vi "ZMQTestSubscriber.vi"() -> ()   [LabVIEW 2017]
uses:
  <vilib>/addons/zeromq/socket_type.ctl
  <vilib>/addons/zeromq/socket_options.ctl
  <vilib>/Analysis/baseanly.llb/Mean (DBL).vi
  <vilib>/addons/zeromq/zmq_context.lvclass
  <vilib>/addons/zeromq/zeromq.lvlib
  <vilib>/addons/zeromq/zmq_socket.lvclass
  <vilib>/Analysis/NI_AALBase.lvlib
panel:
  out "Full event latency std dev":dbl
  out "Full event latency mean":dbl
  out "Short event latency std dev":dbl
  out "Short event latency mean":dbl
  out "Full event latency (ms)":T1(graph)
  out "Short event latency (ms)":T1(graph)
  in  "port":u16=5560
  in  "Stop Button":bool
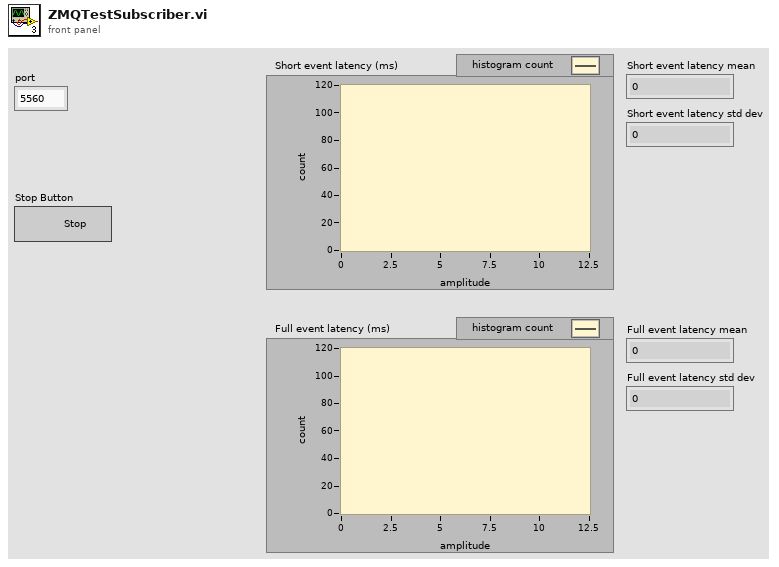
[diagram p1: front panel]
types:
  T1 = cluster{"X Values":dbl[], "Histogram: h(x)":i32[]}
  T2 = typedef "zeromq.lvlib/socket_options.ctl" = enum8{"NONE", "ZMQ_HWM", "<2>", "ZMQ_SWAP", "ZMQ_AFFINITY", "ZMQ_IDENTITY", "ZMQ_SUBSCRIBE", "ZMQ_UNSUBSCRIBE", "ZMQ_RATE", "ZMQ_RECOVERY_IVL", "ZMQ_MCAST_LOOP", "ZMQ_SNDBUF", "ZMQ_RCVBUF", "ZMQ_RCVMORE", "ZMQ_FD", "ZMQ_EVENTS", "ZMQ_TYPE", "ZMQ_LINGER", "ZMQ_RECONNECT_IVL", "ZMQ_BACKLOG", "ZMQ_RECOVERY_IVL_MSEC", "ZMQ_RECONNECT_IVL_MAX", "ZMQ_MAXMSGSIZE", "ZMQ_SNDHWM", "ZMQ_RCVHWM", "ZMQ_MULTICAST_HOPS", "<26>", "ZMQ_RCVTIMEO", "ZMQ_SNDTIMEO", "<29>", "<30>", "ZMQ_IPV4ONLY", "ZMQ_LAST_ENDPOINT", "ZMQ_ROUTER_MANDATORY", "ZMQ_TCP_KEEPALIVE", "ZMQ_TCP_KEEPALIVE_CNT", "ZMQ_TCP_KEEPALIVE_IDLE", "ZMQ_TCP_KEEPALIVE_INTVL", "ZMQ_TCP_ACCEPT_FILTER", "ZMQ_DELAY_ATTACH_ON_CONNECT", "ZMQ_XPUB_VERBOSE"}
  T3 = typedef "zeromq.lvlib/socket_type.ctl" = enum8{"ZMQ_PAIR", "ZMQ_PUB", "ZMQ_SUB", "ZMQ_REQ", "ZMQ_REP", "ZMQ_DEALER", "ZMQ_ROUTER", "ZMQ_PULL", "ZMQ_PUSH", "ZMQ_XPUB", "ZMQ_XSUB"}
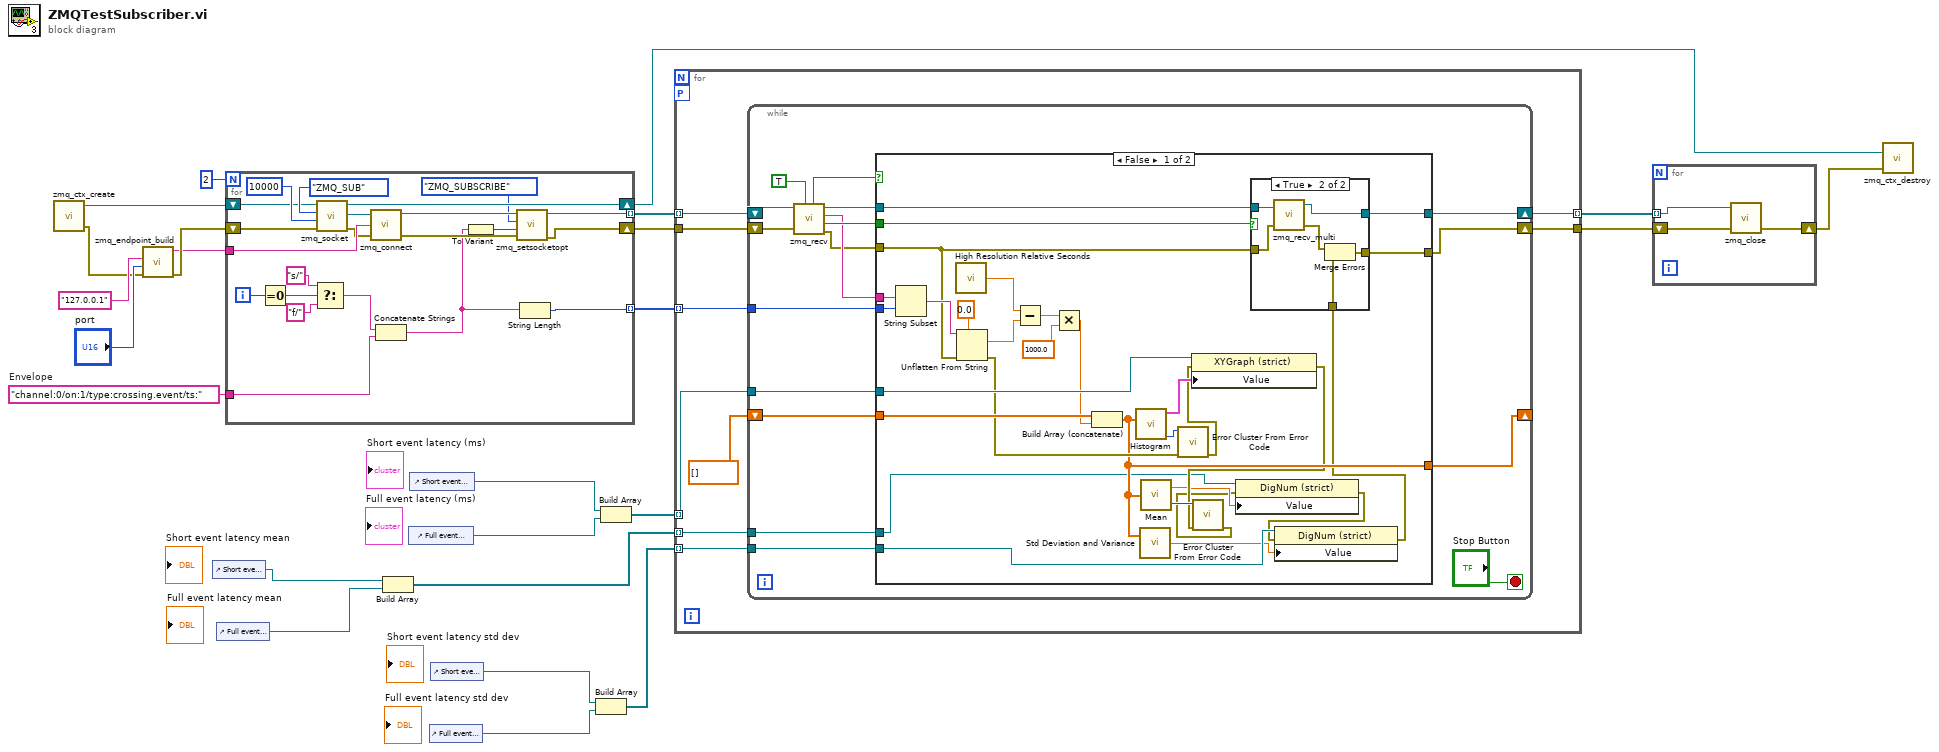
[diagram p0: block diagram]
diagram:
  w16 = "channel:0/on:1/type:crossing.event/ts:"  # Envelope
  n1 = call <vilib>:"zmq_ctx_create.vi"() -> ("error out"=w19:errorcluster, "context out"=w24:refnum<class "zmq_context.lvclass">)  [unwired: 4 in]
  n2 = call <vilib>:"zmq_endpoint_build.vi"("error in"=w19, "port"="port", "address"="127.0.0.1" ("initial string")) -> ("error out"=w18:errorcluster, "endpoint"=w17:string)  [unwired: 2 in, 1 out]
  n3 = control-ref of="Short event latency mean"() -> (w4:refnum<vi>)
  n4 = control-ref of="Full event latency mean"() -> (w3:refnum<vi>)
  n5 = for {
    N: 2 -> [_]
    shift-right: [w42] -> w22
    shift-left: w24 -> [w43]
    shift-right: [w28] -> w15
    shift-left: w18 -> [w44]
    tunnel: w17 -> [w40]
    tunnel: w16 -> [w33]
    tunnel: [w27] -> w13 mode=indexing
    tunnel: [w25] -> w9 mode=indexing
    i -> [w38]
    n6 = Equal To 0?(x=w38) -> (x = 0?=w37:bool)
    n7 = Select(t="s/", s=w37, f="f/") -> (s? t:f=w34:string)
    n8 = call <vilib>:"zmq_socket.vi"("error in"=w44, "linger (ms)"=10000, "socket type"=socket_type."ZMQ_SUB", "context in"=w43) -> ("error out"=w39:errorcluster, "socket out"=w41:refnum<class "zmq_socket.lvclass">, "context out"=w42:refnum<class "zmq_context.lvclass">)  [unwired: 1 in]
    n9 = call <vilib>:"zmq_connect.vi"("error in"=w39, "endpoint"=w40, "socket in"=w41) -> ("error out"=w31:errorcluster, "socket out"=w32:refnum<class "zmq_socket.lvclass">)  [unwired: 1 in]
    n10 = Concatenate Strings(w34, w33) -> (w26:string)
    n11 = To Variant(anything=w26) -> (Variant=w29:variant)
    n12 = call <vilib>:"zmq_setsocketopt.vi"("error in"=w31, "value"=w29, "option"=socket_options."ZMQ_SUBSCRIBE", "socket in"=w32) -> ("error out"=w28:errorcluster, "socket out"=w27:refnum<class "zmq_socket.lvclass">)  [unwired: 2 in]
    n13 = String Length(string=w26) -> (length=w25:i32)
  }
  n14 = Build Array(w4, w3) -> (w2:refnum<vi>[])
  n15 = control-ref of="Full event latency (ms)"() -> (w7:refnum<vi>)
  n16 = control-ref of="Short event latency (ms)"() -> (w8:refnum<vi>)
  n17 = control-ref of="Full event latency std dev"() -> (w5:refnum<vi>)
  n18 = control-ref of="Short event latency std dev"() -> (w6:refnum<vi>)
  n19 = Build Array(w6, w5) -> (w1:refnum<vi>[])
  n20 = Build Array(w8, w7) -> (w10:refnum<vi>[])
  n21 = for {
    tunnel: w13 -> [w53] mode=indexing
    tunnel: [w52] -> w12 mode=indexing
    workers-P: _ -> [_]
    tunnel: w15 -> [w55]
    tunnel: [w54] -> w14
    tunnel: w10 -> [w51] mode=indexing
    tunnel: w9 -> [w50] mode=indexing
    tunnel: w2 -> [w48] mode=indexing
    tunnel: w1 -> [w47] mode=indexing
    n22 = while {
      shift-right: [w60] -> w54
      shift-left: w55 -> [w70]
      shift-right: [w65] -> w52
      shift-left: w53 -> [w69]
      tunnel: w51 -> [w64]
      tunnel: w50 -> [w62]
      shift-right: [w58] -> _
      shift-left: dbl[] [] -> [w59]
      tunnel: w48 -> [w57]
      tunnel: w47 -> [w56]
      stop <- "Stop Button" stop-if-true
      n23 = call <vilib>:"zmq_recv.vi"("no block? (F)"=TRUE, "error in"=w70, "socket in"=w69) -> ("error out"=w61:errorcluster, "more?"=w66:bool, "data"=w63:string, "socket out"=w67:refnum<class "zmq_socket.lvclass">, "timeout?"=w68:bool)  [unwired: 2 in]
      n24 = case shown="False" w68 {
        tunnel: w67 -> [w101 w113]
        tunnel: w66 -> [w102 _]
        tunnel: [w100 w113] -> w65
        tunnel: w64 -> [w99 _]
        tunnel: w63 -> [w97 _]
        tunnel: w62 -> [w98 _]
        tunnel: w61 -> [w90 w112]
        tunnel: [w89 w112] -> w60
        tunnel: w59 -> [w88 w111]
        tunnel: [w81 w111] -> w58
        tunnel: w57 -> [w79 _]
        tunnel: w56 -> [w76 _]
        frame False {
          n25 = String Subset(string=w97, offset (0)=w98) -> (substring=w96:string)  [unwired: 1 in]
          n26 = call <vilib>:"High Resolution Relative Seconds.vi"() -> ("relative seconds"=w94:dbl)
          n27 = Unflatten From String(type=0.0, binary string=w96, error in (no error)=w90) -> (value=w93:dbl, error out=w83:errorcluster)  [unwired: 2 in, 1 out]
          n28 = Subtract(x=w94, y=w93) -> (x-y=w92:dbl)
          n29 = Multiply(x=w92, y=1000.0) -> (x*y=w87:dbl)
          n30 = Build Array (concatenate)(w88, w87) -> (w81:dbl[])
          n31 = call <vilib>:"Histogram.vi"("X"=w81) -> ("error"=w84:i32, "Histogram Graph"=w86:T1)  [unwired: 7 in, 2 out]
          n32 = call <vilib>:"Std Deviation and Variance.vi"("X"=w81) -> ("standard deviation"=w75:dbl)  [unwired: 1 in, 2 out]
          n33 = call-poly <vilib>:"Mean.vi"("X"=w81) -> ("mean"=w78:dbl, "error"=w85:i32)
          n34 = call <vilib>:"Error Cluster From Error Code.vi"("error in (no error)"=w83, "error code (0)"=w84) -> ("error out"=w82:errorcluster)  [unwired: 7 in]
          n35 = property class="XYGraph (strict)"(reference=w99, error in=w82, "Value"=w86) -> (error out=w80:errorcluster)  [unwired: 1 out]
          n36 = call <vilib>:"Error Cluster From Error Code.vi"("error in (no error)"=w80, "error code (0)"=w85) -> ("error out"=w77:errorcluster)  [unwired: 7 in]
          n37 = property class="DigNum (strict)"(reference=w79, error in=w77, "Value"=w78) -> (error out=w74:errorcluster)  [unwired: 1 out]
          n38 = property class="DigNum (strict)"(reference=w76, error in=w74, "Value"=w75) -> (error out=w73:errorcluster)  [unwired: 1 out]
          n39 = case shown="True" w102 {
            tunnel: w101 -> [w104 w110]
            tunnel: [w104 w109] -> w100
            tunnel: w90 -> [_ w108]
            tunnel: [w103 w106] -> w89
            tunnel: w73 -> [w103 w105]
            frame False {
            }
            frame True {
              n40 = call <vilib>:"zmq_recv_multi.vi"("error in"=w108, "socket in"=w110) -> ("error out"=w107:errorcluster, "socket out"=w109:refnum<class "zmq_socket.lvclass">)  [unwired: 1 in, 1 out]
              n41 = Merge Errors(w107, w105) -> (w106:errorcluster)
            }
          }
        }
        frame True {
        }
      }
    }
  }
  n42 = for {
    shift-right: [w115] -> w11
    shift-left: w14 -> [w116]
    tunnel: w12 -> [w114] mode=indexing
    n43 = call <vilib>:"zmq_close.vi"("error in"=w116, "socket"=w114) -> ("error out"=w115:errorcluster)  [unwired: 3 in]
  }
  n44 = call <vilib>:"zmq_ctx_destroy.vi"("error in"=w11, "context in"=w22) -> ()  [unwired: 3 in, 1 out]
